vi "Enable Operator Controls.vi"(8 "error in (no error)":errorcluster, 11 "Enable Disable":T1(ring)) -> (0 "error out":errorcluster)   [LabVIEW 2019]
doc: "Author: Scott Hannahs <sth@magnet.fsu.edu>\nCopyright 2018 Florida State University, All rights reserved."
uses:
  Interlock 32T Net Client Globals.vi
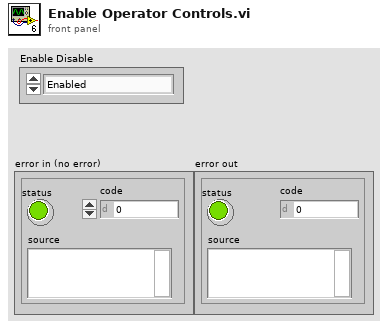
[diagram p1: front panel]
types:
  T1 = enum8{"Enabled", "Disabled", "Disabled and Grayed Out"}
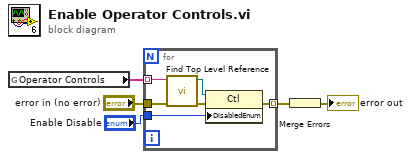
[diagram p0: block diagram]
diagram:
  n1 = global read "Interlock 32T Net Client Globals.vi" "Operator Controls"() -> (w1:string[])
  n2 = for {
    tunnel: "Enable Disable" -> [w10]
    tunnel: w1 -> [w8] mode=indexing
    tunnel: [w7] -> w3 mode=indexing
    tunnel: "error in (no error)" -> [w6]
    n3 = call "Find Top Level Reference.vi"("error in (no error)"=w6, "String"=w8) -> ("error out"=w9:errorcluster, "Ctl Refnum"=w11:refnum<vi>)  [unwired: 8 in]
    n4 = property on="Property Node" class="Ctl"(reference=w11, error in=w9, "DisabledEnum"=w10) -> (error out=w7:errorcluster)  [unwired: 1 out]
  }
  n5 = Merge Errors(w3) -> (→"error out":errorcluster)
